vi "duru1.vi"() -> ()   [LabVIEW 2012]
panel:
  in  "stop":bool
  out "Thermometer":dbl(slide) scale=0.0..100.0
  out "Numeric 2":dbl
  in  "Numeric":dbl
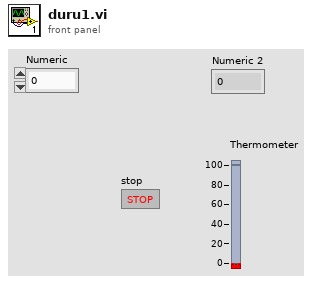
[diagram p1: front panel]
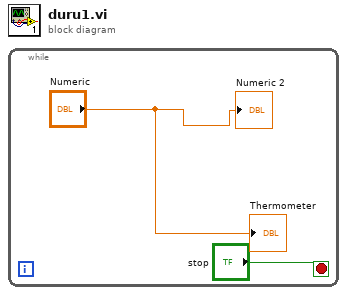
[diagram p0: block diagram]
diagram:
  n1 = while {
    stop <- "stop" stop-if-true
    "Numeric 2" <- "Numeric"
    "Thermometer" <- "Numeric"
  }
